vi "Hough Circle Transform.vi"() -> ()   [LabVIEW 2018]
doc: "Hough Circle Transform: This example is an example of Hough Circle Transform, which considers each pixel in the image as a possible point on the circumference. The goal of the transformation is to find the center coordinates and radii in the accumulator array, which can explain the circles found in the input image."
uses:
  vi.lib/VIRobotics/opencv_yiku/ctls/ColorConversionCodes.ctl
  vi.lib/VIRobotics/opencv_yiku/Mat/Mat_8U/Mat_8U.lvclass
  D:/Program Files/Company/National Instruments/LabVIEW 2018(64bit)/vi.lib/addons/VIRobotics/opencv_yiku/Mat/Mat/Mat.lvclass
  vi.lib/VIRobotics/opencv_yiku/Mat/Create_Mat_8U.vi
  vi.lib/VIRobotics/opencv_yiku/opencv_yiku.lvlib
panel:
  out "gray":picture
  out "circles":picture
  out "circles":cluster{"x":sgl, "y":sgl, "radius":sgl}[](array[cluster])
  in  "parameters":T1={"method"=3, "dp"=1.0, "minDist"=100.0, "param1"=100.0, "param2"=22.0, "minRadius"=30, "maxRadius"=100}
  out "canny":picture
  out "picture":picture
  # "Overview: Demonstrates how to detect circles in an image.\nRequirements: Windows.\nInstructions: \n1.Run the VI"
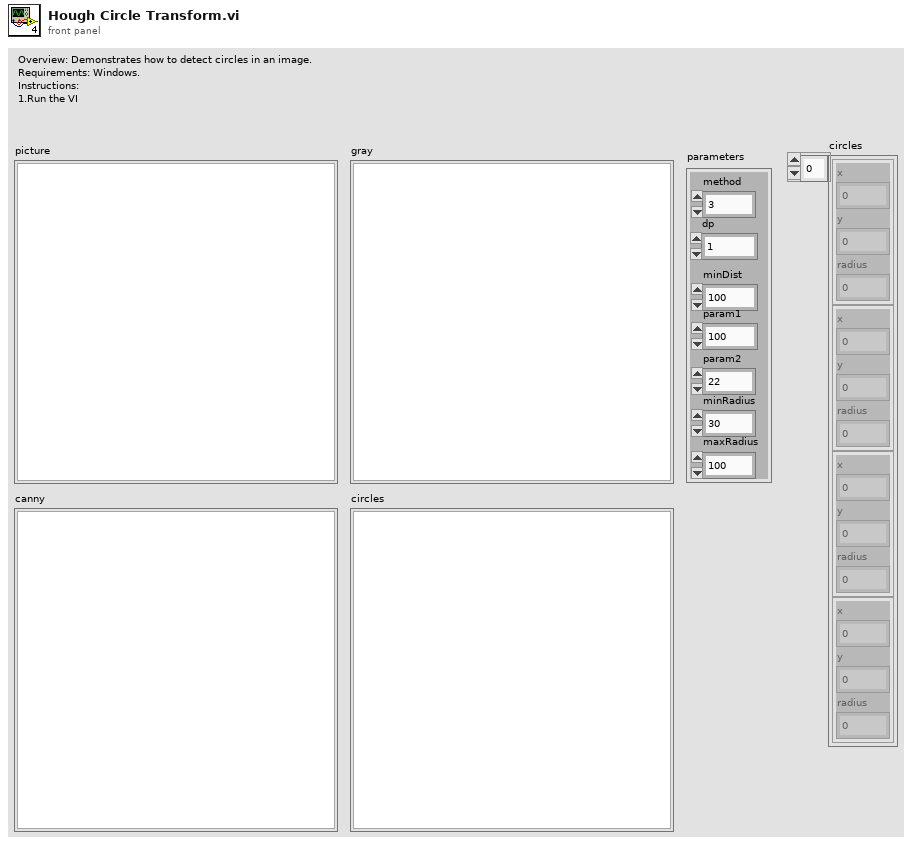
[diagram p1: front panel]
types:
  T1 = cluster{"method":i32, "dp":dbl, "minDist":dbl, "param1":dbl, "param2":dbl, "minRadius":i32, "maxRadius":i32}
  T2 = typedef "opencv_yiku.lvlib/ColorConversionCodes.ctl" = enum32{"COLOR_BGR2BGRA", "COLOR_BGRA2BGR", "COLOR_BGR2RGBA", "COLOR_RGBA2BGR", "COLOR_BGR2RGB", "COLOR_BGRA2RGBA", "COLOR_BGR2GRAY", "COLOR_RGB2GRAY", "COLOR_GRAY2BGR", "COLOR_GRAY2BGRA", "COLOR_BGRA2GRAY", "COLOR_RGBA2GRAY", "COLOR_BGR2BGR565", "COLOR_RGB2BGR565", "COLOR_BGR5652BGR", "COLOR_BGR5652RGB", "COLOR_BGRA2BGR565", "COLOR_RGBA2BGR565", "COLOR_BGR5652BGRA", "COLOR_BGR5652RGBA", "COLOR_GRAY2BGR565", "COLOR_BGR5652GRAY", "COLOR_BGR2BGR555", "COLOR_RGB2BGR555", "COLOR_BGR5552BGR", "COLOR_BGR5552RGB", "COLOR_BGRA2BGR555", "COLOR_RGBA2BGR555", "COLOR_BGR5552BGRA", "COLOR_BGR5552RGBA", "COLOR_GRAY2BGR555", "COLOR_BGR5552GRAY", "COLOR_BGR2XYZ", "COLOR_RGB2XYZ", "COLOR_XYZ2BGR", "COLOR_XYZ2RGB", "COLOR_BGR2YCrCb", "COLOR_RGB2YCrCb", "COLOR_YCrCb2BGR", "COLOR_YCrCb2RGB", "COLOR_BGR2HSV", "COLOR_RGB2HSV", "42", "43", "COLOR_BGR2Lab", "COLOR_RGB2Lab"}
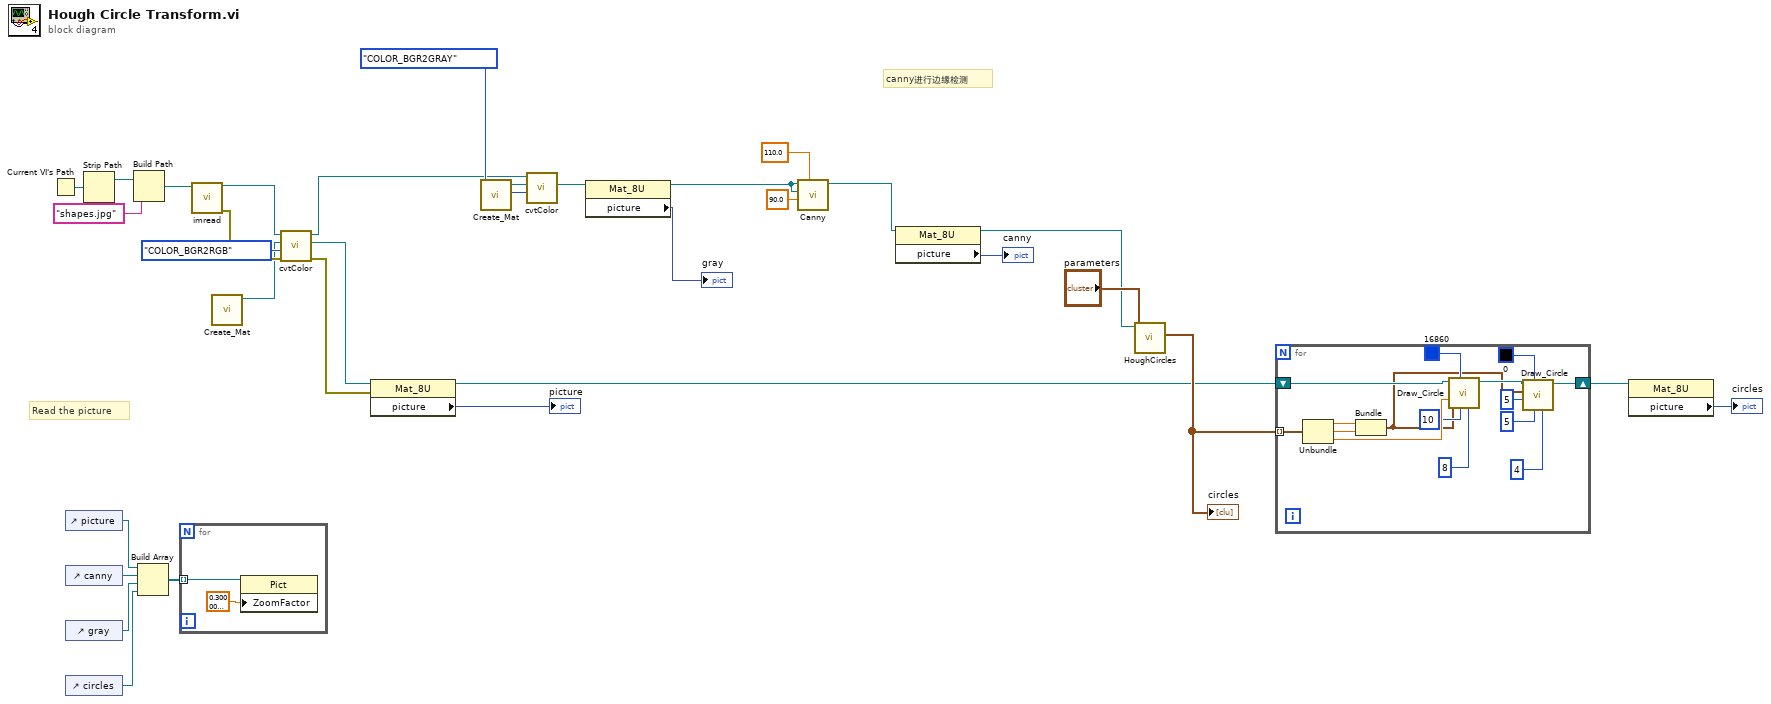
[diagram p0: block diagram]
diagram:
  # "Read the picture"
  # "canny进行边缘检测"
  n1 = Current VI's Path() -> (path=w30:path)
  n2 = control-ref of="picture"() -> (w20:refnum<vi>)
  n3 = control-ref of="canny"() -> (w19:refnum<vi>)
  n4 = control-ref of="gray"() -> (w3:refnum<vi>)
  n5 = control-ref of="circles"() -> (w2:refnum<vi>)
  n6 = Strip Path(path=w30) -> (stripped path=w32:path)  [unwired: 1 out]
  n7 = Build Path(base path=w32, name or relative path="shapes.jpg") -> (appended path=w29:path)
  n8 = Build Array(w20, w19, w3, w2) -> (w18:refnum<vi>[])
  n9 = for {
    tunnel: w18 -> [w34] mode=indexing
    n10 = property class="Pict"(reference=w34, "ZoomFactor"=sgl 0.3 ("Zoom Factor")) -> ()  [unwired: 1 in, 2 out]
  }
  n11 = call "imread.vi"("path"=w29) -> ("error out"=w24:errorcluster, "Mat out"=w25:refnum<class "Mat_8U.lvclass">)  [unwired: 9 in]
  n12 = call-poly "Create_Mat.vi"() -> ("Mat_8U_out"=w13:refnum<class "Mat_8U.lvclass">)  [unwired: 10 in, 1 out]
  n13 = call "cvtColor.vi"("error in (no error)"=w24, "dstCn"=ColorConversionCodes."COLOR_BGR2RGB", "dst"=w13, "src"=w25) -> ("error out"=w23:errorcluster, "dst out"=w12:refnum<class "Mat_8U.lvclass">, "src out"=w11:refnum<class "Mat_8U.lvclass">)  [unwired: 5 in]
  n14 = property class="Mat_8U"(reference=w12, error in=w23) -> (reference out=w10:refnum<class "Mat_8U.lvclass">, "picture"=→"picture":picture)  [unwired: 1 out]
  n15 = call-poly "Create_Mat.vi"() -> ("Mat_8U_out"=w26:refnum<class "Mat_8U.lvclass">)  [unwired: 10 in, 1 out]
  n16 = call "cvtColor.vi"("dstCn"=ColorConversionCodes."COLOR_BGR2GRAY", "dst"=w26, "src"=w11) -> ("dst out"=w1:refnum<class "Mat_8U.lvclass">)  [unwired: 6 in, 2 out]
  n17 = property class="Mat_8U"(reference=w1) -> (reference out=w5:refnum<class "Mat_8U.lvclass">, "picture"=→"gray":picture)  [unwired: 1 in, 1 out]
  n18 = call "Canny.vi"("threshold2"=110.0, "threshold1"=90.0, "dst in"=w5, "Mat in"=w5) -> ("dst out"=w7:refnum<class "Mat_8U.lvclass">)  [unwired: 6 in, 1 out]
  n19 = property class="Mat_8U"(reference=w7) -> (reference out=w6:refnum<class "Mat_8U.lvclass">, "picture"=→"canny":picture)  [unwired: 1 in, 1 out]
  n20 = call "HoughCircles.vi"("parameters"="parameters", "Mat in"=w6) -> ("circles"=w16:cluster{"x":sgl, "y":sgl, "radius":sgl}[])  [unwired: 7 in, 2 out]
  "circles" <- w16
  n21 = for {
    shift-right: [w41] -> w15
    shift-left: w10 -> [w49]
    tunnel: w16 -> [w48] mode=indexing
    n22 = Unbundle(w48) -> ("x"=w47:sgl, "y"=w46:sgl, "radius"=w45:sgl)
    n23 = Bundle("x"=w47, "y"=w46) -> (w38:cluster{"x":sgl, "y":sgl})  [unwired: 1 in]
    n24 = call "Draw_Circle.vi"("lineType"=8, "thickness"=10, "color"=u32 16860, "radius"=w45, "center"=w38, "Mat"=w49) -> ("Mat out"=w42:refnum<class "Mat_8U.lvclass">)  [unwired: 4 in, 1 out]
    n25 = call "Draw_Circle.vi"("lineType"=4, "thickness"=5, "color"=u32 0, "radius"=5, "center"=w38, "Mat"=w42) -> ("Mat out"=w41:refnum<class "Mat_8U.lvclass">)  [unwired: 4 in, 1 out]
  }
  n26 = property class="Mat_8U"(reference=w15) -> ("picture"=→"circles":picture)  [unwired: 1 in, 2 out]
